vi "ifr2025 Close.vi"(8 "error in (no error)":errorcluster, 11 "instrument handle":refnum<visa-resource-name>) -> (0 "error out":errorcluster)   [LabVIEW 2009]
doc: "This VI performs the following operations:\n viClose (instrSession) and\n viClose (rmSession).\n\nNote: The instrument must be re-initialized to use it again."
uses:
  Ifr2025_32.dll
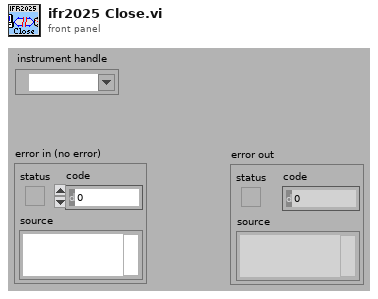
[diagram p1: front panel]
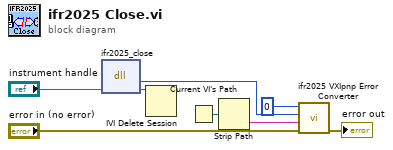
[diagram p0: block diagram]
diagram:
  n1 = dll-call lib="P:/inst/Marconi 2024 Signal Generator/source/labview/ifr2025/ifr2025/ifr2025_*.*" fn="ifr2025_close"("instrument handle"="instrument handle") -> ("status"=w4:i32)  [unwired: 3 in, 3 out]
  n2 = IVI Delete Session(11:"instrument handle") -> ()
  n3 = Current VI's Path() -> (path=w7:path)
  n4 = Strip Path(path=w7) -> (name=w3:string)  [unwired: 1 out]
  n5 = call "ifr2025 VXIpnp Error Converter.vi"("error in (no error)"="error in (no error)", "name of VI (\"\")"=w3, "CVI error code (0)"=w4, "instrument handle"=i8 0) -> ("error out"=→"error out":errorcluster)  [unwired: 7 out]
